vi "Angle 180 to -180.vi"(1 "Angle in":dbl) -> (0 "Angle out":dbl)   [LabVIEW 2023]
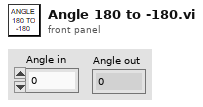
[diagram p1: front panel]
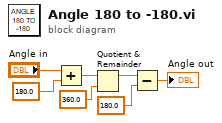
[diagram p0: block diagram]
diagram:
  n1 = Add(x="Angle in", y=180.0) -> (x+y=w5:dbl)
  n2 = Quotient & Remainder(x=w5, y=360.0) -> (x-y*floor(x/y)=w3:dbl)  [unwired: 1 out]
  n3 = Subtract(x=w3, y=180.0) -> (x-y=→"Angle out":dbl)
